vi "Pins to KeySight ENA Sessions.vi"(0 "Semiconductor Module Context":T1, 5 "Pins":string[](array[string]), 11 "error in (no error)":errorcluster) -> (2 "Pin Query Context":refnum<class "MultiplePinMultipleSessionQueryContext.lvclass">, 4 "Semiconductor Module Context Out":T1, 6 "Instrument Sessions":refnum<visa-resource-name>[](array[refnum]), 10 "Channel Lists":string[](array[string]), 15 "error out":errorcluster)   [LabVIEW 2013, in "ENA Custom Instrument.lvlib"]
doc: "Returns NI-VNA sessions required to access one or more pins."
uses:
  ENA Custom Instrument.lvlib
  <vilib>/NI_TestStand_SemiconductorModule/NI_TestStand_Semiconductor_Module.lvlibp/PinMap/General/SemiconductorModuleContext.ctl
  <vilib>/NI_TestStand_SemiconductorModule/NI_TestStand_Semiconductor_Module.lvlibp/PinMap/PinQueryContext/MultiplePinMultipleSessionQueryContext/MultiplePinMultipleSessionQueryContext.lvclass
  <vilib>/NI_TestStand_SemiconductorModule/NI_TestStand_Semiconductor_Module.lvlibp
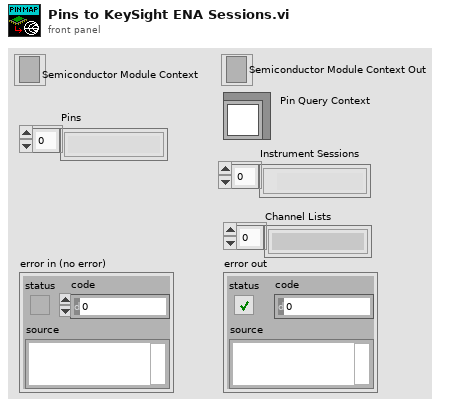
[diagram p1: front panel]
types:
  T1 = typedef "NI_TestStand_Semiconductor_Module.lvlibp/SemiconductorModuleContext.ctl" = refnum<k7>
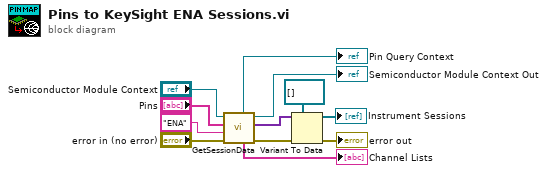
[diagram p0: block diagram]
diagram:
  n1 = call <vilib>:"GetSessionData.vi"("error in (no error)"="error in (no error)", "Instrument Type Id"="ENA", "Pins"="Pins", "Semiconductor Module Context"="Semiconductor Module Context") -> ("error out"=w7:errorcluster, "Session Data"=w6:variant[], "Semiconductor Module Context Out"=→"Semiconductor Module Context Out":T1, "Channel Lists"=→"Channel Lists":string[], "Pin Query Context"=→"Pin Query Context":refnum<class "MultiplePinMultipleSessionQueryContext.lvclass">)  [unwired: 2 in, 1 out]
  n2 = Variant To Data(error in=w7, type=refnum<visa-resource-name>[] [], Variant=w6) -> (data=→"Instrument Sessions":refnum<visa-resource-name>[], error out=→"error out":errorcluster)
